vi "Waypoint Monitor.vi"   [LabVIEW 2011]
uses:
  2 Globals/2 Global.vi
panel:
  # "Waypoint Monitor takes two things from the global variable - the list of waypoints and\nthe position of the robot at the time.\n\nIt compares the current position to the position of the current waypoint, and if that distance\nis less than the required accuracy the current waypoint value is incremented\n\nTODO - Is there a way to only write the Current Waypoint?\nHow do you test something like this that is linked to the global?"
types:
  T1 = typedef "ocuWaypoints.ctl" = cluster{"Waypoints Array":cluster{"Point Type":u16, "Dist/Time":dbl, "UTM Location":T2}[], "Current Waypoint":dbl}
  T2 = typedef "UTM Location.ctl" = cluster{"UTM Zone":dbl, "Hemisphere":enum16{"North", "South"}, "East":dbl, "North":dbl}
  T3 = cluster{"Point Type":u16, "Dist/Time":dbl, "UTM Location":T2}[]
  T4 = cluster{"Point Type":u16, "Dist/Time":dbl, "UTM Location":T2}
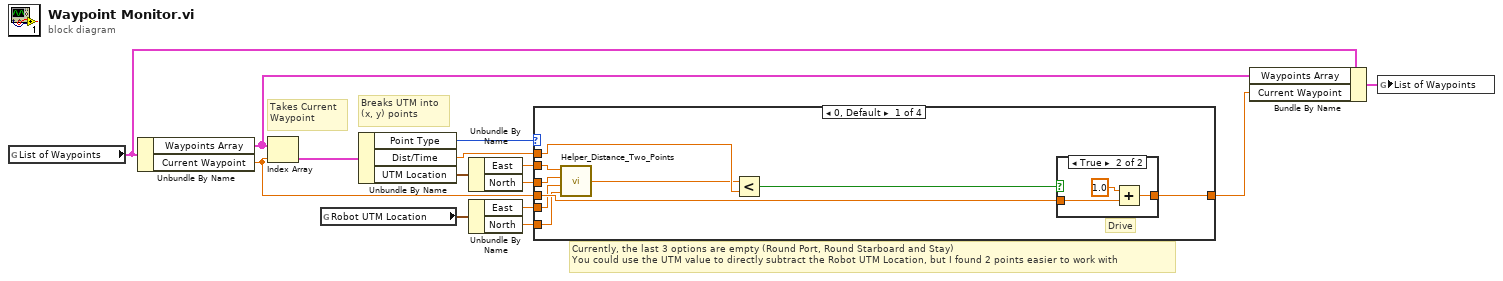
[diagram p0: block diagram]
diagram:
  # "Breaks UTM into\n(x, y) points"
  # "Takes Current\nWaypoint"
  # "Currently, the last 3 options are empty (Round Port, Round Starboard and Stay)\nYou could use the UTM value to directly subtract the Robot UTM Location, but I found 2 points easier to work with"
  n1 = global read "2 Global.vi" "List of Waypoints"() -> (w7:T1)
  n2 = Unbundle By Name(w7) -> ("Waypoints Array"=w11:T3, "Current Waypoint"=w8:dbl)
  n3 = Index Array(array=w11, index=w8) -> (element=w14:T4)
  n4 = global read "2 Global.vi" "Robot UTM Location"() -> (w5:T2)
  n5 = Unbundle By Name(w14) -> ("Point Type"=w13:u16, "Dist/Time"=w12:dbl, "UTM Location"=w6:T2)
  n6 = Unbundle By Name(w6) -> ("East"=w2:dbl, "North"=w1:dbl)
  n7 = Unbundle By Name(w5) -> ("East"=w4:dbl, "North"=w3:dbl)
  n8 = case shown="0, Default" w13 {
    tunnel: w12 -> [w23 _ _ _]
    tunnel: [w20 w28 w29 w30] -> w9
    tunnel: w8 -> [w21 w28 w29 w30]
    tunnel: w4 -> [w16 _ _ _]
    tunnel: w3 -> [w15 _ _ _]
    tunnel: w2 -> [w18 _ _ _]
    tunnel: w1 -> [w17 _ _ _]
    frame 0, Default {
      # "Drive"
      n9 = call "Helper_Distance_Two_Points.vi"("y 2"=w15, "x 2"=w16, "y"=w17, "x"=w18) -> ("Numeric"=w19:dbl)
      n10 = Less?(x=w19, y=w23) -> (x < y?=w22:bool)
      n11 = case shown="True" w22 {
        tunnel: w21 -> [w24 w27]
        tunnel: [w24 w25] -> w20
        frame False {
        }
        frame True {
          n12 = Add(x=1.0, y=w27) -> (x+y=w25:dbl)
        }
      }
    }
    frame 1 {
      # "Round Port"
    }
    frame 2 {
      # "Round Starboard"
    }
    frame 3 {
      # "Stay"
    }
  }
  n13 = Bundle By Name(cluster=w7, "Waypoints Array"=w11, "Current Waypoint"=w9) -> (w10:T1)
  n14 = global write "2 Global.vi" "List of Waypoints"(w10) -> ()
